vi "Autonomous Independent.vi"() -> ()   [LabVIEW 2018]
doc: "This VI is called when autonomous begins, and will automatically be terminated when autonomous ends. You can carry out timed or sensor driven robot movement independently without needing to return to the caller."
uses:
  <vilib>/Rock Robotics/Network Tables/NT Read String Array.vi
  Swerve/SwerveGlobals.vi
  <vilib>/addons/control/pid/pid.llb/PID (DBL).vi
  <vilib>/addons/control/pid/NI_PID_pid.lvlib
panel:
  in  "PID gains":T1={"proportional gain (Kc)"=1.0, "integral time (Ti, min)"=0.01, "derivative time (Td, min)"=0.0} {"derivative time (Td, min)" format="%.3f"; "integral time (Ti, min)" format="%.3f"; "proportional gain (Kc)" format="%.3f"}
  # "Be sure to right-click and choose Data Operations>>Make Current Value default if you want to save the array values with the VI"
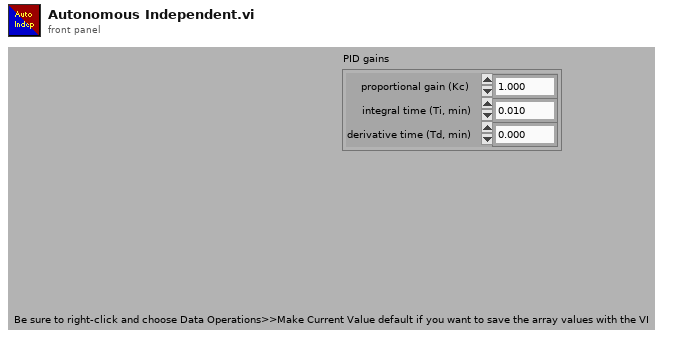
[diagram p1: front panel]
types:
  T1 = cluster{"proportional gain (Kc)":dbl, "integral time (Ti, min)":dbl, "derivative time (Td, min)":dbl}
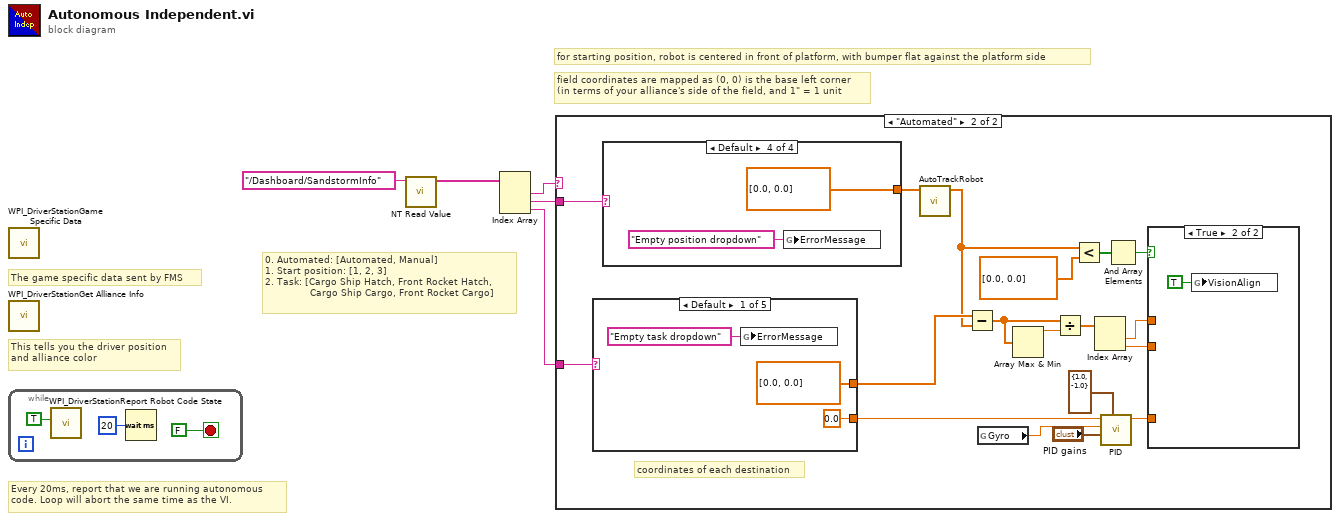
[diagram p0: block diagram]
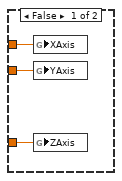
[diagram p3: hidden frame]
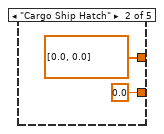
[diagram p4: hidden frame]
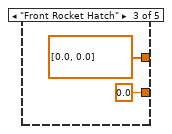
[diagram p5: hidden frame]
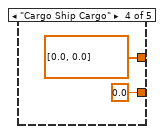
[diagram p6: hidden frame]
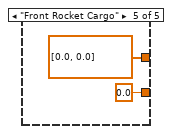
[diagram p7: hidden frame]
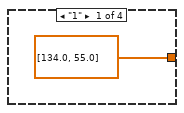
[diagram p8: hidden frame]
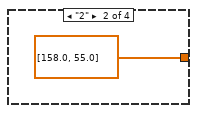
[diagram p9: hidden frame]
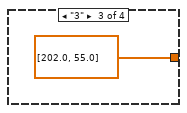
[diagram p10: hidden frame]
diagram:
  # "for starting position, robot is centered in front of platform, with bumper flat against the platform side"
  # "field coordinates are mapped as (0, 0) is the base left corner\n(in terms of your alliance's side of the field, and 1\" = 1 unit"
  # "0. Automated: [Automated, Manual]\n1. Start position: [1, 2, 3]\n2. Task: [Cargo Ship Hatch, Front Rocket Hatch,\n               Cargo Ship Cargo, Front Rocket Cargo]"
  # "The game specific data sent by FMS"
  # "Every 20ms, report that we are running autonomous\ncode. Loop will abort the same time as the VI."
  # "This tells you the driver position\nand alliance color"
  n1 = call <vilib>:"WPI_DriverStationGame Specific Data.vi"() -> ()  [unwired: 11 in, 1 out]
  n2 = call <vilib>:"WPI_DriverStationGet Alliance Info.vi"() -> ()  [unwired: 12 out]
  n3 = while {
    stop <- FALSE stop-if-true
    n4 = call <vilib>:"WPI_DriverStationReport Robot Code State.vi"("Autonomous"=TRUE) -> ()  [unwired: 10 in, 1 out]
    n5 = Wait (ms)(milliseconds to wait=u32 20) -> ()  [unwired: 1 out]
  }
  n6 = call-poly <vilib>:"NT Read Value.vi"("Name"="/Dashboard/SandstormInfo") -> ("String Array"=w4:string[])  [unwired: 9 in, 1 out]
  n7 = Index Array(array=w4) -> (element #1=w2:string, element #2=w3:string, element #3=w1:string)  [unwired: 3 in]
  n8 = case shown="\"Automated\"" w2 {
    tunnel: w3 -> [_ w25]
    tunnel: w1 -> [_ w24]
    frame "Manual", Default {
    }
    frame "Automated" {
      # "coordinates of each destination"
      n9 = case shown="Default" w24 {
        tunnel: [dbl[] [0.0, 0.0] ("Destination (x, y)") dbl[] [0.0, 0.0] ("Destination (x, y)") dbl[] [0.0, 0.0] ("Destination (x, y)") dbl[] [0.0, 0.0] ("Destination (x, y)") dbl[] [0.0, 0.0] ("Destination (x, y)")] -> w23
        tunnel: [0.0 ("Destination (angle)") 0.0 ("Destination (angle)") 0.0 ("Destination (angle)") 0.0 ("Destination (angle)") 0.0 ("Destination (angle)")] -> w17
        frame Default {
          n10 = global write "SwerveGlobals.vi" "ErrorMessage"("Empty task dropdown" ("ErrorMessage")) -> ()
        }
        frame "Cargo Ship Hatch" {
        }
        frame "Front Rocket Hatch" {
        }
        frame "Cargo Ship Cargo" {
        }
        frame "Front Rocket Cargo" {
        }
      }
      n11 = case shown="Default" w25 {
        tunnel: [dbl[] [134.0, 55.0] dbl[] [158.0, 55.0] dbl[] [202.0, 55.0] dbl[] [0.0, 0.0]] -> w26
        frame "1" {
        }
        frame "2" {
        }
        frame "3" {
        }
        frame Default {
          n12 = global write "SwerveGlobals.vi" "ErrorMessage"("Empty position dropdown" ("ErrorMessage")) -> ()
        }
      }
      n13 = call "AutoTrackRobot.vi"("StartCoordinates"=w26) -> ("Coordinates"=w9:dbl[])  [unwired: 10 in]
      n14 = Subtract(x=w23, y=w9) -> (x-y=w22:dbl[])
      n15 = global read "SwerveGlobals.vi" "Gyro"() -> (w14:dbl)
      n16 = Array Max & Min(array=w22) -> (max value=w21:dbl)  [unwired: 3 out]
      n17 = Divide(x=w22, y=w21) -> (x/y=w20:dbl[])
      n18 = Less?(x=w9, y=dbl[] [0.0, 0.0]) -> (x < y?=w11:bool[])
      n19 = Index Array(array=w20) -> (element #1=w19:dbl, element #2=w18:dbl)  [unwired: 2 in]
      n20 = call-poly <vilib>:"PID.vi"("output range"=cluster{"output high":dbl, "output low":dbl} {"output high"=1.0, "output low"=-1.0}, "PID gains"="PID gains", "process variable"=w14, "setpoint"=w17) -> ("output"=w16:dbl)  [unwired: 6 in, 1 out]
      n21 = And Array Elements(Boolean array=w11) -> (logical AND=w10:bool)
      n22 = case shown="True" w10 {
        tunnel: w19 -> [w29 _]
        tunnel: w18 -> [w28 _]
        tunnel: w16 -> [w27 _]
        frame False {
          n23 = global write "SwerveGlobals.vi" "XAxis"(w29) -> ()
          n24 = global write "SwerveGlobals.vi" "YAxis"(w28) -> ()
          n25 = global write "SwerveGlobals.vi" "ZAxis"(w27) -> ()
        }
        frame True {
          n26 = global write "SwerveGlobals.vi" "VisionAlign"(TRUE ("VisionAlign")) -> ()
        }
      }
    }
  }
